vi "12-2.vi"() -> ()   [LabVIEW 2019, in "12.lvlib"]
uses:
  12.lvlib
  e1706d2a-1850-4533-9028-034c938844d6.vi
panel:
  out "size(s)":i32[](array[numeric])
  out "Routes out":string[][](array[string])
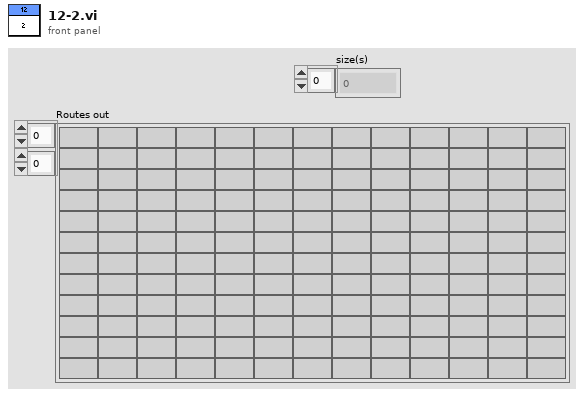
[diagram p1: front panel]
types:
  T1 = cluster{"Cave":string, "Small(F)/Big(T)":bool, "Remaining Visits":i32, "Connected Caves":string[]}
  T2 = cluster{"Cave":string, "Small(F)/Big(T)":bool, "Remaining Visits":i32, "Connected Caves":string[]}[]
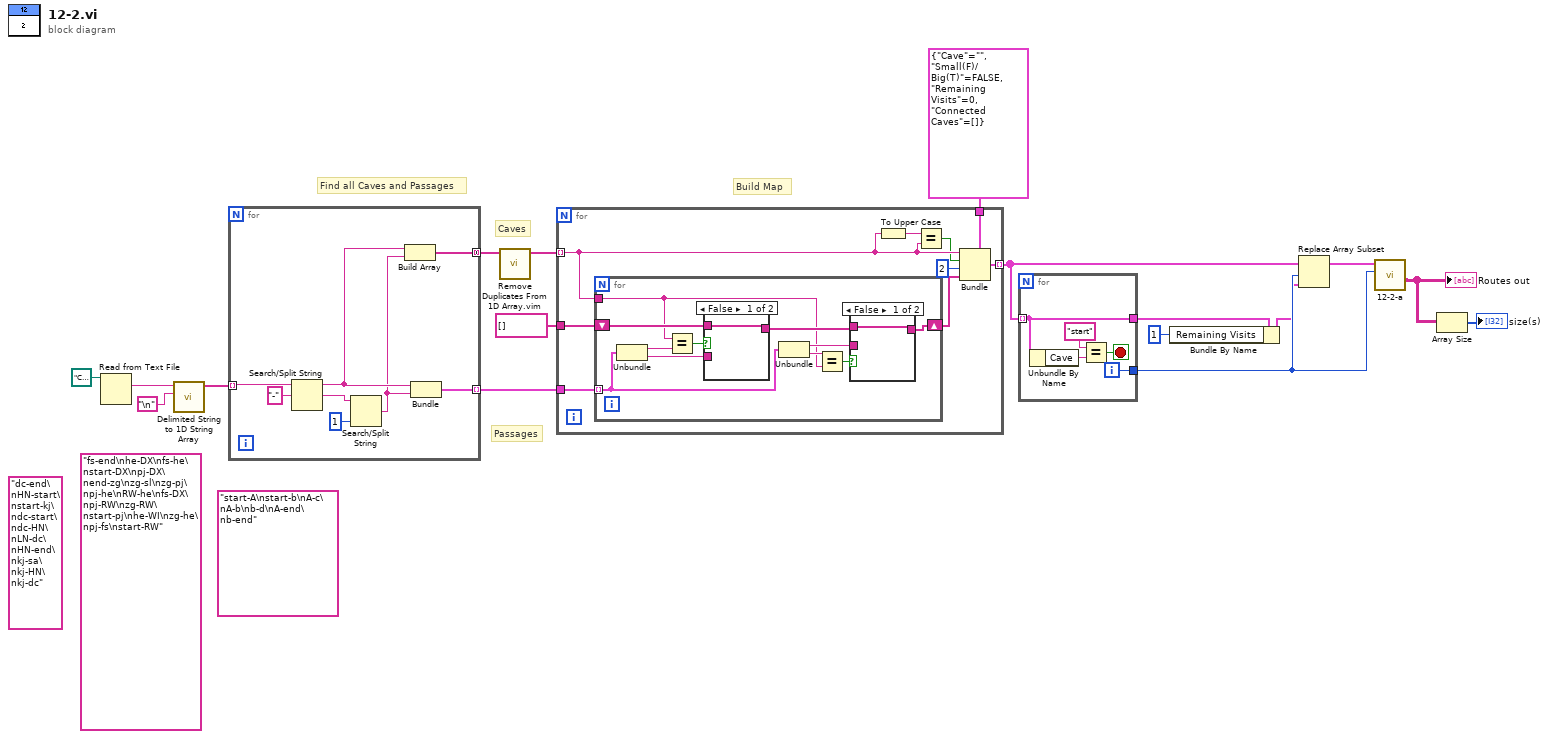
[diagram p0: block diagram]
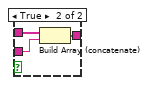
[diagram p2: hidden frame]
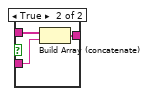
[diagram p3: hidden frame]
diagram:
  (unwired) "fs-end\nhe-DX\nfs-he\nstart-DX\npj-DX\nend-zg\nzg-sl\nzg-pj\npj-he\nRW-he\nfs-DX\npj-RW\nzg-RW\nstart-pj\nhe-WI\nzg-he\npj-fs\nstart-RW"
  (unwired) "dc-end\nHN-start\nstart-kj\ndc-start\ndc-HN\nLN-dc\nHN-end\nkj-sa\nkj-HN\nkj-dc"
  (unwired) "start-A\nstart-b\nA-c\nA-b\nb-d\nA-end\nb-end"
  # "Build Map"
  # "Find all Caves and Passages"
  # "Passages"
  # "Caves"
  n1 = Read from Text File(file (use dialog)=path "C:/Users/craig.walker/Documents/GitHub/lv2019-Advent-of-Code-2021/12/input.txt") -> (text=w1:string)  [unwired: 3 in, 3 out]
  n2 = call <vilib>:"Delimited String to 1D String Array.vi"("delimiter"="\n", "delimited string"=w1) -> ("string array"=w16:string[])  [unwired: 9 in]
  n3 = for {
    tunnel: w16 -> [w25] mode=indexing
    tunnel: [w20] -> w15 mode=concatenating
    tunnel: [w18] -> w13 mode=indexing
    n4 = Search/Split String(string=w25, search string/char (-)="-") -> (substring before match=w23:string, match + rest of string=w22:string)  [unwired: 1 in, 1 out]
    n5 = Search/Split String(string=w22, offset (0)=1) -> (match + rest of string=w19:string)  [unwired: 1 in, 2 out]
    n6 = Build Array(w23, w19) -> (w20:string[])
    n7 = Bundle("String"=w23, "String"=w19) -> (w18:cluster{"String":string, "String":string})  [unwired: 1 in]
  }
  n8 = call "Remove Duplicates From 1D Array.vim"("array"=w15) -> ("array with duplicates removed"=w14:string[])  [unwired: 10 in]
  n9 = for {
    tunnel: w14 -> [w30] mode=indexing
    tunnel: w13 -> [w34]
    tunnel: string[] [] -> [w33]
    tunnel: T1 {"Cave"="", "Small(F)/Big(T)"=FALSE, "Remaining Visits"=0, "Connected Caves"=[]} ("cluster") -> [w28]
    tunnel: [w27] -> w8 mode=indexing
    n10 = for {
      tunnel: w34 -> [w36] mode=indexing
      tunnel: w30 -> [w37]
      shift-right: [w35] -> w32
      shift-left: w33 -> [w43]
      n11 = Unbundle(w36) -> ("String"=w44:string, "String"=w42:string)
      n12 = Equal?(x=w37, y=w44) -> (x = y?=w45:bool)
      n13 = case shown="False" w45 {
        tunnel: w43 -> [w50 w53]
        tunnel: w42 -> [_ w52]
        tunnel: [w50 w51] -> w41
        frame False {
        }
        frame True {
          n14 = Build Array (concatenate)(w53, w52) -> (w51:string[])
        }
      }
      n15 = Unbundle(w36) -> ("String"=w39:string, "String"=w38:string)
      n16 = Equal?(x=w38, y=w37) -> (x = y?=w40:bool)
      n17 = case shown="False" w40 {
        tunnel: w41 -> [w46 w49]
        tunnel: w39 -> [_ w48]
        tunnel: [w46 w47] -> w35
        frame False {
        }
        frame True {
          n18 = Build Array (concatenate)(w49, w48) -> (w47:string[])
        }
      }
    }
    n19 = To Upper Case(1:w30) -> (0:w31:string)
    n20 = Equal?(x=w31, y=w30) -> (x = y?=w29:bool)
    n21 = Bundle(cluster=w28, "Cave"=w30, "Small(F)/Big(T)"=w29, "Remaining Visits"=2, "Connected Caves"=w32) -> (w27:T1)
  }
  n22 = for {
    tunnel: w8 -> [w54] mode=indexing
    tunnel: [w55] -> w5
    tunnel: [w54] -> w4
    i -> [w55]
    stop <- w56 stop-if-true
    n23 = Unbundle By Name(w54) -> ("Cave"=w58:string)
    n24 = Equal?(x="start", y=w58) -> (x = y?=w56:bool)
  }
  n25 = Bundle By Name(cluster=w4, "Remaining Visits"=1) -> (w3:T1)
  n26 = Replace Array Subset(array=w8, new element=w3, index=w5) -> (w6:T2)
  n27 = call "12-2-a.vi"("Start Index"=w5, "Array"=w6) -> ("Route out"=w7:string[][])  [unwired: 9 in]
  "Routes out" <- w7
  n28 = Array Size(array=w7) -> (size(s)=→"size(s)":i32[])
